vi "求均值.vi"(10 "采样次数":dbl, 11 "散斑图像作用结果优化":dbl[](array[numeric])) -> (3 "均值":dbl)   [LabVIEW 2018]
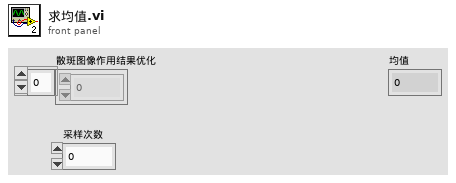
[diagram p1: front panel]
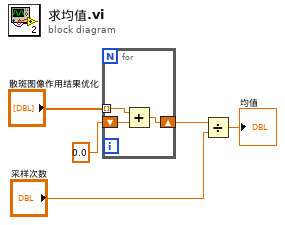
[diagram p0: block diagram]
diagram:
  n1 = for {
    shift-right: [w7] -> w2
    shift-left: 0.0 -> [w6]
    tunnel: "散斑图像作用结果优化" -> [w8] mode=indexing
    n2 = Add(x=w8, y=w6) -> (x+y=w7:dbl)
  }
  n3 = Divide(x=w2, y="采样次数") -> (x/y=→"均值":dbl)
